vi "Read FunctionIniFilePath.vi"(8 "error in (no error)":errorcluster, 11 "Sim_Ideal_PMU in":refnum<class "Sim_Ideal_PMU.lvclass">) -> (0 "error out":errorcluster, 2 "FunctionIniFilePath":string, 3 "Sim_Ideal_PMU out":refnum<class "Sim_Ideal_PMU.lvclass">)   [LabVIEW 2018, in "SensorPlugins.lvlib" / "Sim_Ideal_PMU.lvclass"]
uses:
  Sim_Ideal_PMU.lvclass
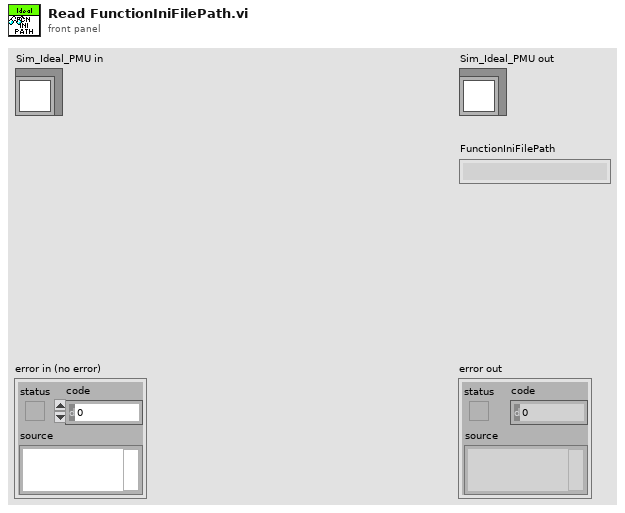
[diagram p1: front panel]
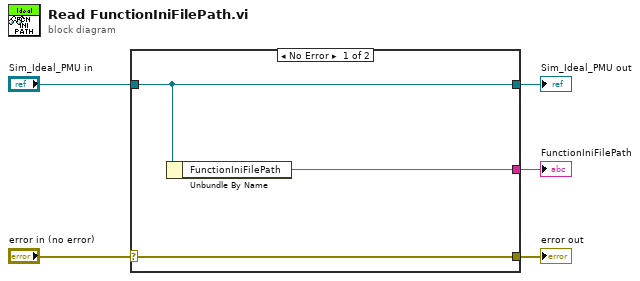
[diagram p0: block diagram]
diagram:
  n1 = case shown="No Error" "error in (no error)" {
    selector: "error in (no error)" -> [w8 w9]
    tunnel: [w8 w9] -> w4
    tunnel: [w7 w10] -> w2
    tunnel: "Sim_Ideal_PMU in" -> [w7 w10]
    tunnel: [w6 _] -> w1
    frame No Error {
      n2 = Unbundle By Name(w7) -> ("FunctionIniFilePath"=w6:string)
    }
    frame Error {
    }
  }
  "error out" <- w4
  "Sim_Ideal_PMU out" <- w2
  "FunctionIniFilePath" <- w1
